vi "Read Active measurements enqueuers.vi"(8 "error in (no error)":errorcluster, 11 "Measure Controller in":refnum<class "Process Controller.lvclass">) -> (0 "error out":errorcluster, 2 "Active measurements enqueuers":refnum<class "Message Enqueuer.lvclass">[](array[class]), 3 "Measure Controller out":refnum<class "Process Controller.lvclass">)   [LabVIEW 2016, in "Process Controller.lvclass"]
uses:
  Process Controller.lvclass
  <vilib>/ActorFramework/Message Enqueuer/Message Enqueuer.lvclass
  Process Controller.lvclass/Process Controller.ctl
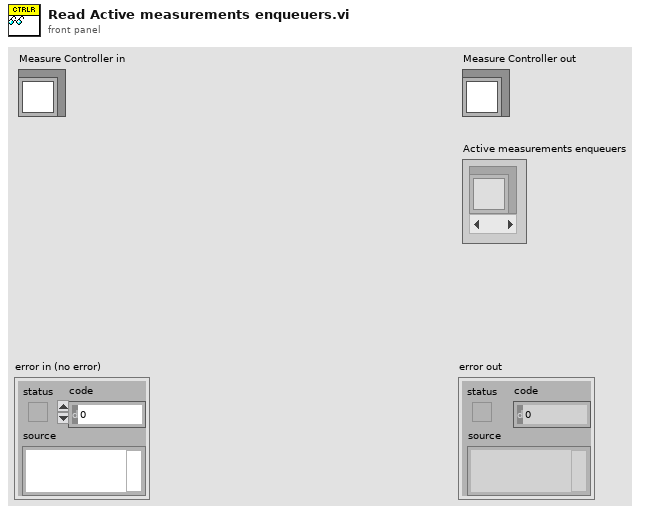
[diagram p1: front panel]
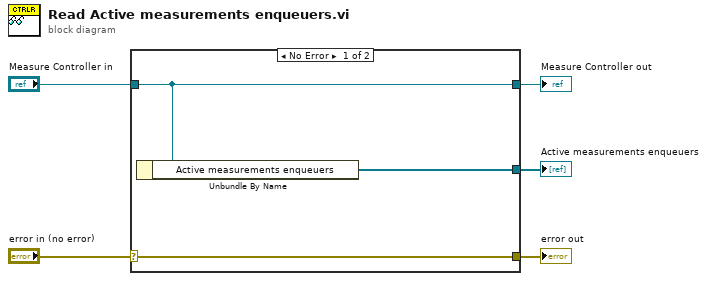
[diagram p0: block diagram]
diagram:
  n1 = case shown="No Error" "error in (no error)" {
    selector: "error in (no error)" -> [w8 w9]
    tunnel: [w8 w9] -> w4
    tunnel: [w7 w10] -> w2
    tunnel: "Measure Controller in" -> [w7 w10]
    tunnel: [w6 _] -> w1
    frame No Error {
      n2 = Unbundle By Name(w7) -> ("Active measurements enqueuers"=w6:refnum<class "Message Enqueuer.lvclass">[])
    }
    frame Error {
    }
  }
  "error out" <- w4
  "Measure Controller out" <- w2
  "Active measurements enqueuers" <- w1
